vi "Config ALC Search Span.vi"(0 "VISA Resource Name":refnum<visa-resource-name>, 1 "State (F: OFF)":bool, 2 "Span Type  (0: Full)":enum16{"Full", "User"}(ring) format="%.0g", 3 "Start (0.0)":dbl, 4 "Stop (0.0)":dbl, 5 "error in (no error)":errorcluster {"code" format="%.0x"}) -> (14 "VISA Resource Name Out":refnum<visa-resource-name>, 19 "error out":errorcluster {"code" format="%.0x"})   [LabVIEW 2014, in "Agilent ESG Series.lvlib"]
doc: "This VI configures span power search subsystem.\n\nNotes:\n(1) This VI is supported for Agilent E4438C only."
uses:
  Agilent ESG Series.lvlib
panel:
  # "ON"
  # "OFF"
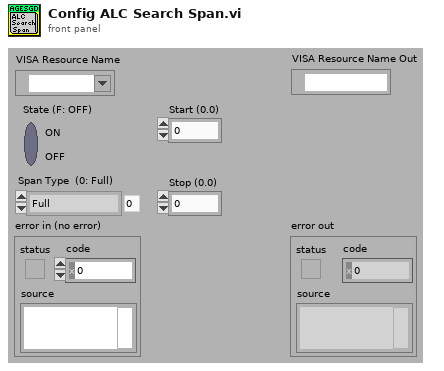
[diagram p1: front panel]
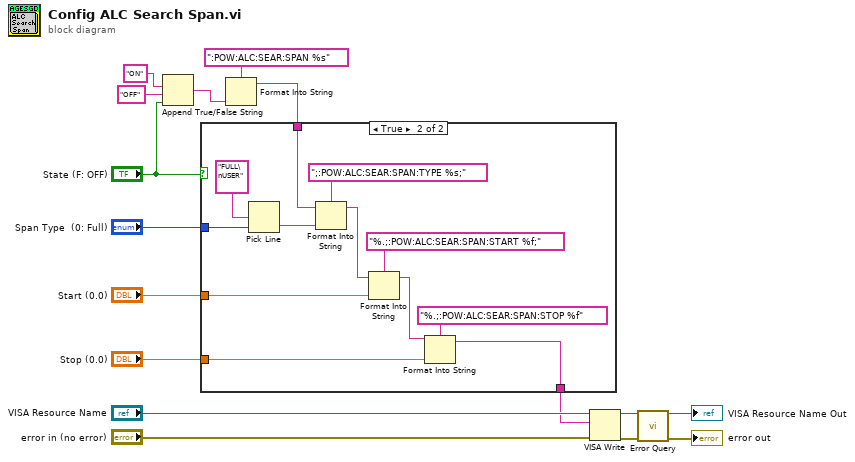
[diagram p0: block diagram]
diagram:
  n1 = Append True/False String(1:"State (F: OFF)", 2:"OFF" ("false string"), 3:"ON" ("multi-line string")) -> (0:w5:string)  [unwired: 1 in]
  n2 = Format Into String(format string=":POW:ALC:SEAR:SPAN %s", w5) -> (resulting string=w4:string)  [unwired: 2 in, 1 out]
  n3 = case shown="True" "State (F: OFF)" {
    tunnel: "Start (0.0)" -> [_ w28]
    tunnel: "Stop (0.0)" -> [_ w26]
    tunnel: "Span Type  (0: Full)" -> [_ w22]
    tunnel: w4 -> [w17 w21]
    tunnel: [w17 w20] -> w3
    frame False {
    }
    frame True {
      n4 = Pick Line(multi-line string="FULL\nUSER", line index=w22) -> (output string=w23:string)  [unwired: 1 in]
      n5 = Format Into String(format string=";:POW:ALC:SEAR:SPAN:TYPE %s;", initial string=w21, w23) -> (resulting string=w19:string)  [unwired: 1 in, 1 out]
      n6 = Format Into String(format string="%.;:POW:ALC:SEAR:SPAN:START %f;", initial string=w19, w28) -> (resulting string=w18:string)  [unwired: 1 in, 1 out]
      n7 = Format Into String(format string="%.;:POW:ALC:SEAR:SPAN:STOP %f", initial string=w18, w26) -> (resulting string=w20:string)  [unwired: 1 in, 1 out]
    }
  }
  n8 = VISA Write(VISA resource name="VISA Resource Name", write buffer=w3, error in (no error)="error in (no error)") -> (VISA resource name out=w12:refnum<visa-resource-name>, error out=w11:errorcluster)  [unwired: 1 out]
  n9 = call "Error Query.vi"("VISA Resource Name"=w12, "error in (no error)"=w11) -> ("VISA Resource Name Out"=→"VISA Resource Name Out":refnum<visa-resource-name>, "error out"=→"error out":errorcluster)  [unwired: 10 in, 2 out]
